vi "Rectangle size and position to bounds.vi"(10 "Position":T4, 11 "Size":T3 {"Y" format="%.3f"; "X" format="%.3f"}) -> (2 "bounds with rot":T1 {"angle" format="%.3f"; "bottom" format="%.3f"; "right" format="%.3f"; "top" format="%.3f"; "left" format="%.3f"}, 3 "bounds":T2 {"bottom" format="%.3f"; "right" format="%.3f"; "top" format="%.3f"; "left" format="%.3f"})   [LabVIEW 2023]
doc: "For some controls, the bounds are returned as areas, and the position is returned as the top-left position. This VI converts these values into a standard top-left-bottom-right bounds cluster.\n\nPositon: Left, Top\nSize: Width, Height\n\nThe output with rotation is useful for ROI functions in Vision. Will always be zero."
uses:
  <vilib>/Utility/miscctls.llb/LVPositionTypeDef.ctl
  Controls/x,y cluster_DBL.ctl
  Controls/Rect or Line Cluster.ctl
  Controls/Rect with angle Cluster.ctl
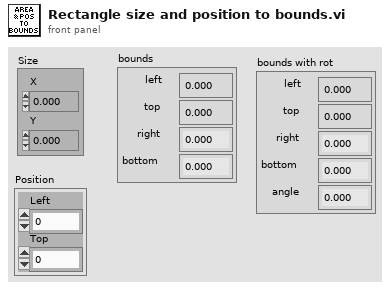
[diagram p1: front panel]
types:
  T1 = typedef "Rect with angle Cluster.ctl" = cluster{"left":dbl, "top":dbl, "right":dbl, "bottom":dbl, "angle":dbl}
  T2 = typedef "Rect or Line Cluster.ctl" = cluster{"left":dbl, "top":dbl, "right":dbl, "bottom":dbl}
  T3 = typedef "x,y cluster_DBL.ctl" = cluster{"X":dbl, "Y":dbl}
  T4 = typedef "LVPositionTypeDef.ctl" = cluster{"Left":i32, "Top":i32}
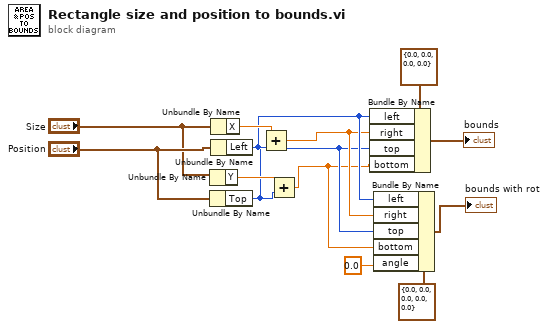
[diagram p0: block diagram]
diagram:
  n1 = Unbundle By Name("Size") -> ("Y"=w13:dbl)
  n2 = Unbundle By Name("Position") -> ("Top"=w5:i32)
  n3 = Unbundle By Name("Size") -> ("X"=w10:dbl)
  n4 = Unbundle By Name("Position") -> ("Left"=w7:i32)
  n5 = Add(x=w10, y=w7) -> (x+y=w6:dbl)
  n6 = Add(x=w13, y=w5) -> (x+y=w4:dbl)
  n7 = Bundle By Name(cluster=T2 {"left"=0.0, "top"=0.0, "right"=0.0, "bottom"=0.0} ("bounds"), "left"=w7, "right"=w6, "top"=w5, "bottom"=w4) -> (→"bounds":T2)
  n8 = Bundle By Name(cluster=T1 {"left"=0.0, "top"=0.0, "right"=0.0, "bottom"=0.0, "angle"=0.0} ("bounds with rot"), "left"=w7, "right"=w6, "top"=w5, "bottom"=w4, "angle"=0.0 ("Rotation")) -> (→"bounds with rot":T1)
